vi "SimpleOscillograph.vi"() -> ()   [LabVIEW 2015]
uses:
  <vilib>/Analysis/4window.llb/Hanning Window (DBL).vi
  <vilib>/Analysis/4window.llb/Hamming Window (DBL).vi
  <vilib>/Analysis/4window.llb/Blackman Window (DBL).vi
  <vilib>/Analysis/4window.llb/Gaussian Window (DBL).vi
  <vilib>/Analysis/2dsp.llb/Real FFT.vi
  <vilib>/Analysis/4window.llb/AllCosWindow (DBL).vi
  <vilib>/Instr/_visa.llb/VISA Configure Serial Port (Serial Instr).vi
  <vilib>/Analysis/NI_AALPro.lvlib
panel:
  out "AD":i32
  out "VCC":dbl
  out "num_of_data":i32
  out "实际采样频率":dbl
  in  "采样模式":u16(ring) items=["触发", "实时"]
  in  "ABORT":bool
  in  "触发模式":u16(ring) items=["自动", "上升沿", "下降沿", "边沿"]
  in  "采 样 率":u16(ring)=3 caption="端口号" items=["100Hz", "1KHz", "10KHz", "100KHz", "250KHz", "500KHz", "1MHz"]
  in  "清空缓冲区":bool
  in  "清空波形":bool
  out "C1":dbl
  out "C2":dbl
  out "C3":dbl
  out "缓冲区字节":u32
  in  "波特率":u16(ring)=4 items=["4800", "9600", "115200", "230400", "460800"]
  out "串口状态":bool
  in  "打开串口":bool
  in  "端口号":u16(ring) items=["COM1", "COM2", "COM3", "COM4", "COM5", "COM6"]
  in  "?":enum32{"独立波形图", "混合波形图", "FFT频域图"}(tab)
  out "幅值 C3":dbl(graph)
  out "幅值 C2":dbl(graph)
  out "幅值 C1":dbl(graph)
  out "幅值":dynamicdata(graph)
  in  "FIR滤波":u16(ring) caption="端口号" items=["禁用"]
  in  "信号加窗":u16(ring) caption="端口号" items=["不加窗", "Hanning", "Hamming", "Blackman", "高斯窗"]
  in  "FFT通道":u16(ring) caption="端口号" items=["C1", "C2", "C3"]
  out "频谱图":dbl[](graph)
  out "关串口等待":u32=500
  in  "延时":u32
  out "VISA resource name":refnum<visa-resource-name> caption="VISA资源名称"
  # "SimpleOscillograph"
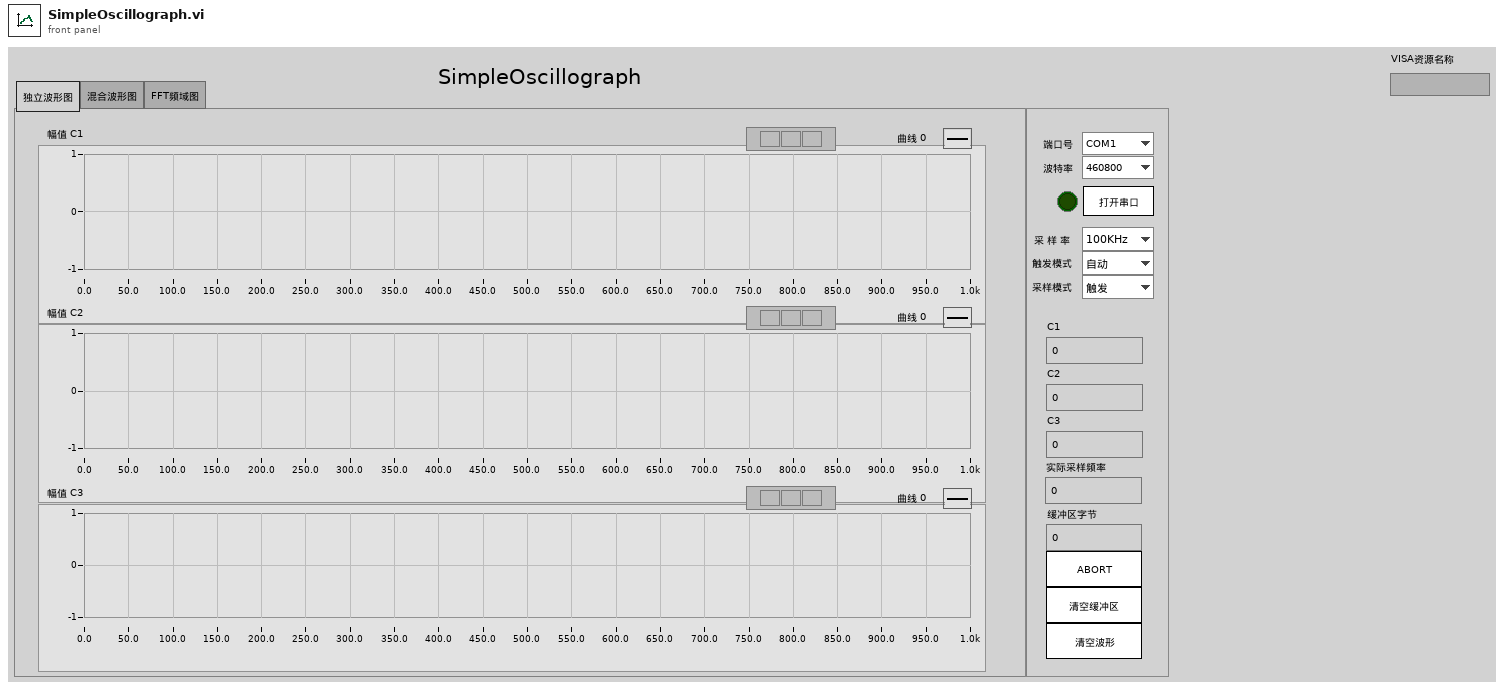
[diagram p1: front panel]
types:
  T1 = enum8{"Enabled", "Disabled", "Disabled and Grayed Out"}
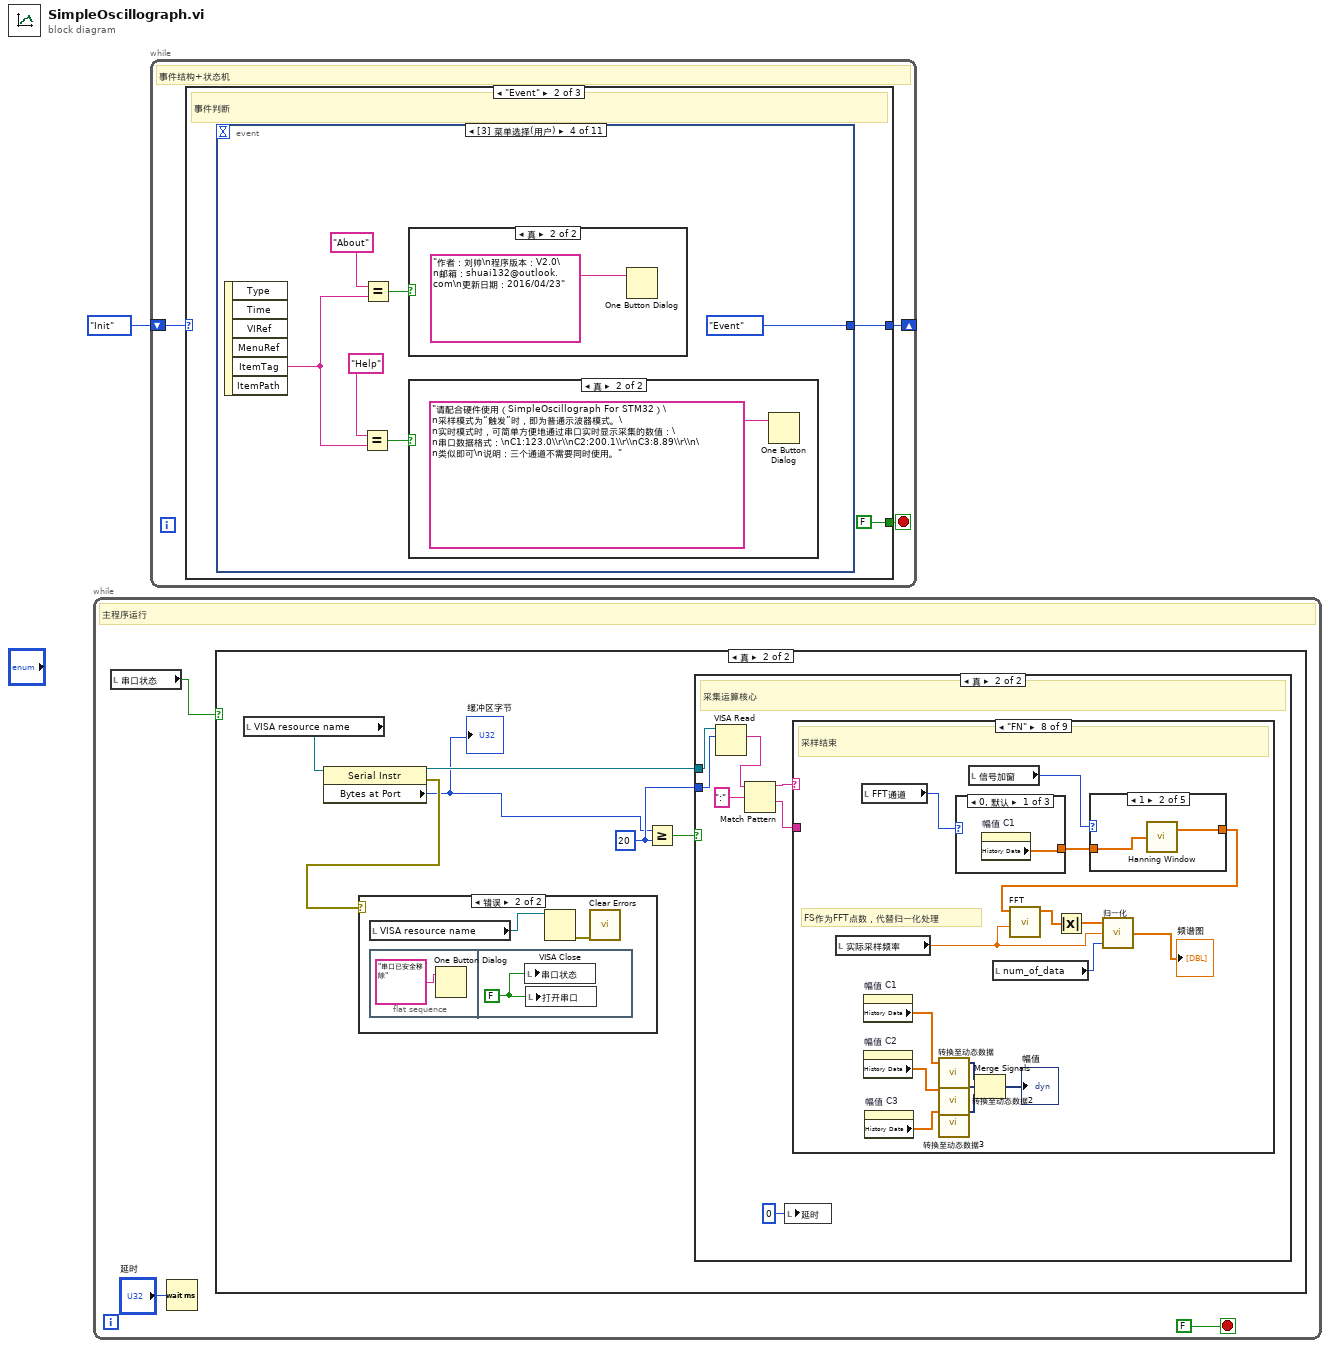
[diagram p0: block diagram]
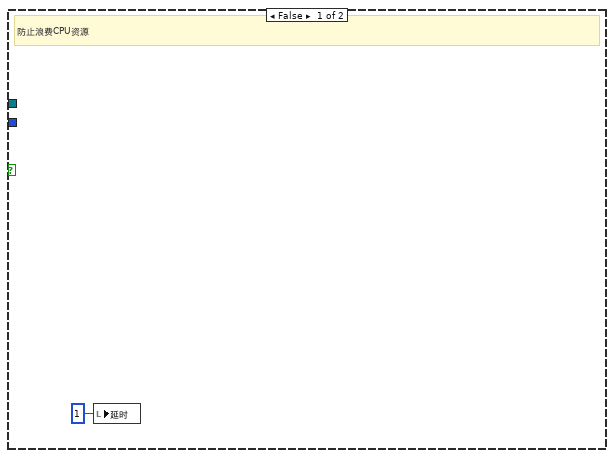
[diagram p4: hidden frame]
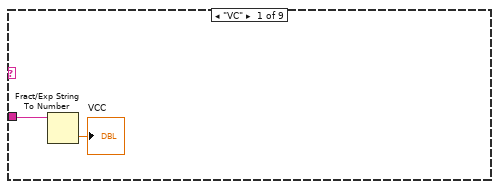
[diagram p5: hidden frame]
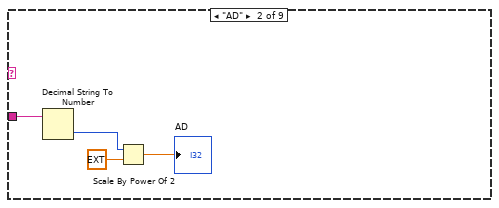
[diagram p6: hidden frame]
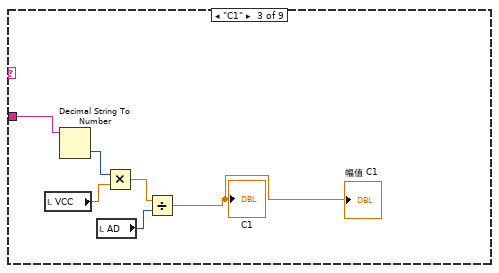
[diagram p7: hidden frame]
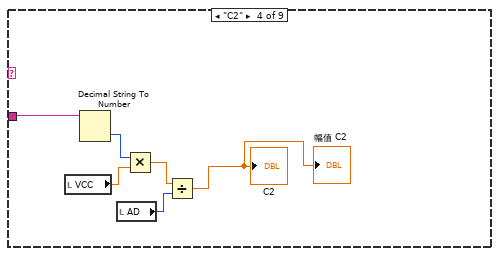
[diagram p8: hidden frame]
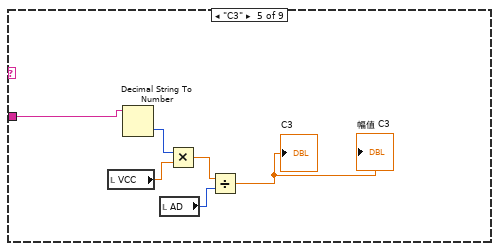
[diagram p9: hidden frame]
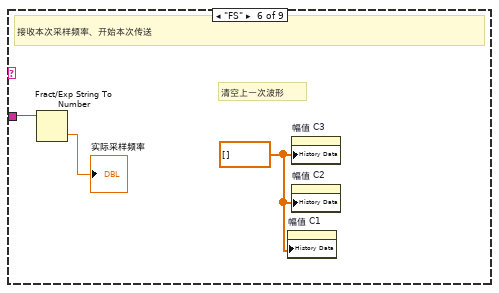
[diagram p10: hidden frame]
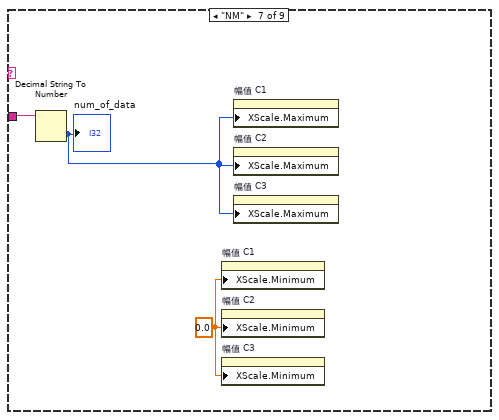
[diagram p11: hidden frame]
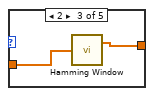
[diagram p13: hidden frame]
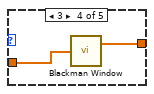
[diagram p14: hidden frame]
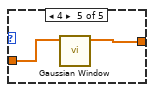
[diagram p15: hidden frame]
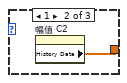
[diagram p16: hidden frame]
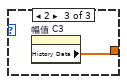
[diagram p17: hidden frame]
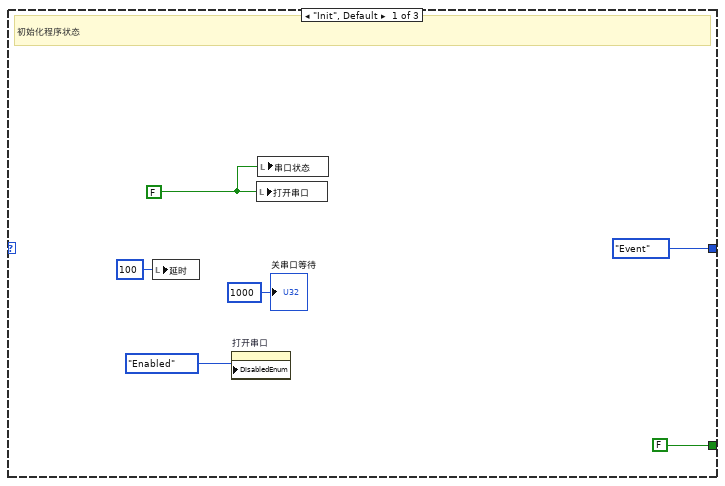
[diagram p19: hidden frame]
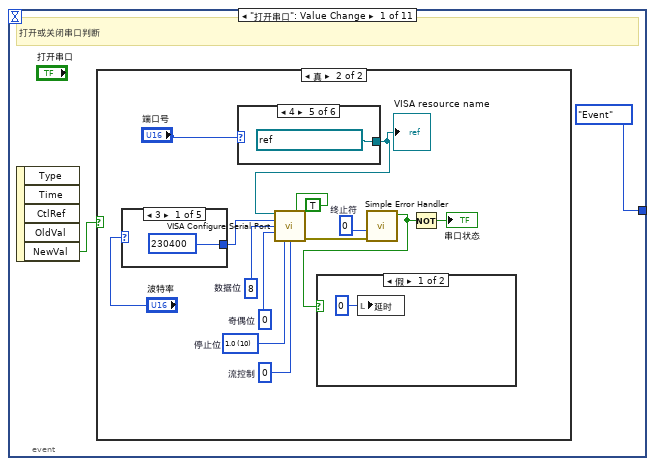
[diagram p20: hidden frame]
diagram:
  n1 = while {
    stop <- FALSE stop-if-true
    # "主程序运行"
    n2 = local read "串口状态"() -> (w4:bool)
    n3 = Wait (ms)(milliseconds to wait="延时") -> ()  [unwired: 1 out]
    n4 = case shown="真" w4 {
      frame False {
      }
      frame True {
        w6 = u32 20 ("y")
        n5 = local read "VISA resource name"() -> (w10:refnum<visa-resource-name>)
        n6 = property class="Serial Instr"(reference=w10) -> (reference out=w9:refnum<visa-resource-name>, error out=w8:errorcluster, "Bytes at Port"=w5:u32)  [unwired: 1 in]
        "缓冲区字节" <- w5
        n7 = case shown="错误" w8 {
          frame No Error {
          }
          frame Error {
            n8 = local read "VISA resource name"() -> (w11:refnum<visa-resource-name>)
            n9 = flat-sequence {
              frame #0 {
                n10 = One Button Dialog(message="串口已安全移除") -> ()  [unwired: 1 in, 1 out]
              }
              frame #1 {
                w14 = FALSE ("exit")
                n11 = local write "串口状态"(w14) -> ()
                n12 = local write "打开串口"(w14) -> ()
              }
            }
            n13 = VISA Close(VISA resource name=w11) -> (error out=w12:errorcluster)  [unwired: 1 in]
            n14 = call <vilib>:"Clear Errors.vi"("error in (no error)"=w12) -> ()  [unwired: 5 in, 2 out]
          }
        }
        n15 = Greater Or Equal?(x=w5, y=w6) -> (x >= y?=w7:bool)
        n16 = case shown="真" w7 {
          tunnel: w9 -> [_ w22]
          tunnel: w6 -> [_ w21]
          frame False {
            # "防止浪费CPU资源"
            n17 = local write "延时"(u32 1 ("延时")) -> ()
          }
          frame True {
            # "采集运算核心"
            n18 = VISA Read(VISA resource name=w22, byte count=w21) -> (read buffer=w16:string)  [unwired: 1 in, 3 out]
            n19 = Match Pattern(string=w16, regular expression=":" ("正则表达式")) -> (before substring=w18:string, after substring=w19:string)  [unwired: 1 in, 2 out]
            n20 = local write "延时"(u32 0 ("延时")) -> ()
            n21 = case shown="\"FN\"" w18 {
              tunnel: w19 -> [w24 w28 w34 w36 w42 w49 w52 _ _]
              frame "VC" {
                n22 = Fract/Exp String To Number(string=w24) -> (number=→"VCC":dbl)  [unwired: 3 in, 1 out]
              }
              frame "AD" {
                n23 = Decimal String To Number(string=w28) -> (number=w27:i32)  [unwired: 2 in, 1 out]
                n24 = Scale By Power Of 2(n=w27, x=ext 1.0) -> (x*2^n=→"AD":ext)
              }
              frame "C1" {
                n25 = local read "VCC"() -> (w32:dbl)
                n26 = Decimal String To Number(string=w34) -> (number=w33:i32)  [unwired: 2 in, 1 out]
                n27 = local read "AD"() -> (w30:i32)
                n28 = Multiply(x=w33, y=w32) -> (x*y=w31:dbl)
                n29 = Divide(x=w31, y=w30) -> (x/y=→"C1" →"幅值 C1":dbl)
              }
              frame "C2" {
                n30 = local read "VCC"() -> (w39:dbl)
                n31 = Decimal String To Number(string=w36) -> (number=w40:i32)  [unwired: 2 in, 1 out]
                n32 = local read "AD"() -> (w37:i32)
                n33 = Multiply(x=w40, y=w39) -> (x*y=w38:dbl)
                n34 = Divide(x=w38, y=w37) -> (x/y=→"C2" →"幅值 C2":dbl)
              }
              frame "C3" {
                n35 = local read "VCC"() -> (w45:dbl)
                n36 = Decimal String To Number(string=w42) -> (number=w46:i32)  [unwired: 2 in, 1 out]
                n37 = local read "AD"() -> (w43:i32)
                n38 = Multiply(x=w46, y=w45) -> (x*y=w44:dbl)
                n39 = Divide(x=w44, y=w43) -> (x/y=→"C3" →"幅值 C3":dbl)
              }
              frame "FS" {
                w47 = dbl[] [] ("历史数据")
                # "清空上一次波形"
                # "接收本次采样频率、开始本次传送"
                n40 = Fract/Exp String To Number(string=w49) -> (number=→"实际采样频率":dbl)  [unwired: 3 in, 1 out]
                n41 = property on="幅值 C1" class="WFChart (严格)"("History Data"=w47) -> ()  [unwired: 2 in, 2 out]
                n42 = property on="幅值 C3" class="WFChart (严格)"("History Data"=w47) -> ()  [unwired: 2 in, 2 out]
                n43 = property on="幅值 C2" class="WFChart (严格)"("History Data"=w47) -> ()  [unwired: 2 in, 2 out]
              }
              frame "NM" {
                w50 = 0.0 ("X标尺.范围:最小值")
                n44 = Decimal String To Number(string=w52) -> (number=w51:i32)  [unwired: 2 in, 1 out]
                "num_of_data" <- w51
                n45 = property on="幅值 C1" class="WFChart (严格)"("XScale.Minimum"=w50) -> ()  [unwired: 2 in, 2 out]
                n46 = property on="幅值 C2" class="WFChart (严格)"("XScale.Minimum"=w50) -> ()  [unwired: 2 in, 2 out]
                n47 = property on="幅值 C3" class="WFChart (严格)"("XScale.Minimum"=w50) -> ()  [unwired: 2 in, 2 out]
                n48 = property on="幅值 C1" class="WFChart (严格)"("XScale.Maximum"=w51) -> ()  [unwired: 2 in, 2 out]
                n49 = property on="幅值 C2" class="WFChart (严格)"("XScale.Maximum"=w51) -> ()  [unwired: 2 in, 2 out]
                n50 = property on="幅值 C3" class="WFChart (严格)"("XScale.Maximum"=w51) -> ()  [unwired: 2 in, 2 out]
              }
              frame "FN" {
                # "FS作为FFT点数，代替归一化处理"
                # "采样结束"
                n51 = local read "实际采样频率"() -> (w62:dbl)
                n52 = local read "FFT通道"() -> (w68:u16)
                n53 = property on="幅值 C1" class="WFChart (严格)"() -> ("History Data"=w59:dbl[])  [unwired: 2 in, 2 out]
                n54 = property on="幅值 C2" class="WFChart (严格)"() -> ("History Data"=w57:dbl[])  [unwired: 2 in, 2 out]
                n55 = property on="幅值 C3" class="WFChart (严格)"() -> ("History Data"=w55:dbl[])  [unwired: 2 in, 2 out]
                n56 = call "转换至动态数据"("Array"=w59) -> ("Dynamic Data Type"=w58:dynamicdata)  [unwired: 3 in]
                n57 = call "转换至动态数据2"("Array"=w57) -> ("Dynamic Data Type"=w56:dynamicdata)  [unwired: 3 in]
                n58 = call "转换至动态数据3"("Array"=w55) -> ("Dynamic Data Type"=w54:dynamicdata)  [unwired: 3 in]
                n59 = case shown="0, 默认" w68 {
                  tunnel: [w78 w79 w80] -> w67
                  frame 0, Default {
                    n60 = property on="幅值 C1" class="WFChart (严格)"() -> ("History Data"=w78:dbl[])  [unwired: 2 in, 2 out]
                  }
                  frame 1 {
                    n61 = property on="幅值 C2" class="WFChart (严格)"() -> ("History Data"=w79:dbl[])  [unwired: 2 in, 2 out]
                  }
                  frame 2 {
                    n62 = property on="幅值 C3" class="WFChart (严格)"() -> ("History Data"=w80:dbl[])  [unwired: 2 in, 2 out]
                  }
                }
                n63 = local read "信号加窗"() -> (w66:u16)
                n64 = Merge Signals(w58, w56, w54) -> (→"幅值":dynamicdata)
                n65 = local read "num_of_data"() -> (w60:i32)
                n66 = case shown="1" w66 {
                  tunnel: w67 -> [w69 w71 w73 w75 w77]
                  tunnel: [w69 w70 w72 w74 w76] -> w64
                  frame 0, Default {
                  }
                  frame 1 {
                    n67 = call-poly <vilib>:"Hanning Window.vi"("X"=w71) -> ("Windowed X"=w70:dbl[])  [unwired: 1 out]
                  }
                  frame 2 {
                    n68 = call-poly <vilib>:"Hamming Window.vi"("X"=w73) -> ("Windowed X"=w72:dbl[])  [unwired: 1 out]
                  }
                  frame 3 {
                    n69 = call-poly <vilib>:"Blackman Window.vi"("X"=w75) -> ("Windowed X"=w74:dbl[])  [unwired: 1 out]
                  }
                  frame 4 {
                    n70 = call-poly <vilib>:"Gaussian Window.vi"("X"=w77) -> ("Windowed X"=w76:dbl[])  [unwired: 9 in, 1 out]
                  }
                }
                n71 = call-poly <vilib>:"FFT.vi"("FFT size"=w62, "X"=w64) -> ("FFT {X}"=w65:cdb[])  [unwired: 8 in, 1 out]
                n72 = Absolute Value(x=w65) -> (abs(x)=w63:dbl[])
                n73 = call "归一化.vi"("实际参采样点数"=w60, "FFT点数"=w62, "数组输入"=w63) -> ("数组输出"=→"频谱图":dbl[])
              }
              frame Default {
              }
            }
          }
        }
      }
    }
  }
  n74 = while {
    shift-right: [w81] -> _
    shift-left: enum16{"Init", "Event", "Exit"}."Init" -> [w82]
    stop <- w83 stop-if-true
    # "事件结构+状态机"
    n75 = case shown="\"Event\"" w82 {
      tunnel: [FALSE FALSE TRUE] -> w83
      tunnel: [enum16{"Init", "Event", "Exit"}."Event" w90 enum16{"Init", "Event", "Exit"}."Exit"] -> w81
      frame "Init", Default {
        w87 = FALSE ("exit")
        # "初始化程序状态"
        n76 = local write "延时"(u32 100 ("延时")) -> ()
        n77 = property on="打开串口" class="Bool (严格)"("DisabledEnum"=T1."Enabled" ("禁用")) -> ()  [unwired: 2 in, 2 out]
        n78 = local write "打开串口"(w87) -> ()
        n79 = local write "串口状态"(w87) -> ()
        "关串口等待" <- u32 1000 ("关串口等待")
      }
      frame "Event" {
        # "事件判断"
        n80 = event shown="[3] 菜单选择(用户)" {
          selector: _ -> [_ _ _ _ _ _ _ _ _ _ _]
          dyn-events: _ -> [_ _ _ _ _ _ _ _ _ _ _]
          timeout: _ -> [_ _ _ _ _ _ _ _ _ _ _]
          tunnel: [enum16{"Init", "Event", "Exit"}."Event" enum16{"Init", "Event", "Exit"}."Event" enum16{"Init", "Event", "Exit"}."Event" enum16{"Init", "Event", "Exit"}."Event" enum16{"Init", "Event", "Exit"}."Event" enum16{"Init", "Event", "Exit"}."Event" enum16{"Init", "Event", "Exit"}."Event" enum16{"Init", "Event", "Exit"}."Event" enum16{"Init", "Event", "Exit"}."Event" enum16{"Init", "Event", "Exit"}."Event" enum16{"Init", "Event", "Exit"}."Exit"] -> w90
          event "打开串口": Value Change {
            # "打开或关闭串口判断"
            n81 = event-data() -> ("NewVal"=w92:bool)  [unwired: 1 in, 4 out]
            n82 = case shown="真" w92 {
              frame False {
                n83 = local read "串口状态"() -> (w94:bool)
                n84 = case shown="真" w94 {
                  frame False {
                  }
                  frame True {
                    # "故意先关串口状态\n这样主程序就不会占用串口了\n降低出错的可能"
                    n85 = flat-sequence {
                      frame #0 {
                        n86 = local write "串口状态"(FALSE) -> ()
                        n87 = local write "延时"(u32 100 ("延时")) -> ()
                      }
                      frame #1 {
                        n88 = local read "VISA resource name"() -> (w97:refnum<visa-resource-name>)
                        n89 = VISA Close(VISA resource name=w97) -> (error out=w98:errorcluster)  [unwired: 1 in]
                        n90 = call <vilib>:"Simple Error Handler.vi"("error in (no error)"=w98) -> ()  [unwired: 4 in, 5 out]
                      }
                      frame #2 {
                        n91 = local read "关串口等待"() -> (w99:u32)
                        n92 = Wait (ms)(milliseconds to wait=w99) -> ()  [unwired: 1 out]
                      }
                    }
                  }
                }
              }
              frame True {
                w100 = u16 10 items=["1.0"=10, "1.5"=15, "2.0"=20]  # 停止位
                w104 = TRUE  # 终止符
                w110 = u16 0  # 流控制
                w109 = u8 0  # 奇偶位
                w108 = u16 8  # 数据位
                n93 = case shown="3" "波特率" {
                  tunnel: [230400 460800 4800 9600 115200] -> w107
                  frame 3 {
                  }
                  frame 4 {
                  }
                  frame 0, Default {
                  }
                  frame 1 {
                  }
                  frame 2 {
                  }
                }
                n94 = case shown="4" "端口号" {
                  tunnel: [refnum<visa-resource-name> "ASRL1::INSTR" ("VISA resource name") refnum<visa-resource-name> "ASRL2::INSTR" ("VISA resource name") refnum<visa-resource-name> "ASRL3::INSTR" ("VISA resource name") refnum<visa-resource-name> "ASRL4::INSTR" ("VISA resource name") refnum<visa-resource-name> "ASRL5::INSTR" ("VISA resource name") refnum<visa-resource-name> "ASRL6::INSTR" ("VISA resource name")] -> w101
                  frame 0, Default {
                  }
                  frame 1 {
                  }
                  frame 2 {
                  }
                  frame 3 {
                  }
                  frame 4 {
                  }
                  frame 5 {
                  }
                }
                "VISA resource name" <- w101
                n95 = call-poly "VISA Configure Serial Port"("VISA resource name"=w101, "Enable Termination\nChar (T)"=w104, "baud rate (9600)"=w107, "data bits (8)"=w108, "parity (0:none)"=w109, "stop bits (10: 1 bit)"=w100, "flow control (0:none)"=w110) -> ("error out"=w111:errorcluster)  [unwired: 7 in, 1 out]
                n96 = call <vilib>:"Simple Error Handler.vi"("type of dialog (OK msg:1)"=0, "error in (no error)"=w111) -> ("error?"=w105:bool)  [unwired: 3 in, 4 out]
                n97 = case shown="假" w105 {
                  frame False {
                    n98 = local write "延时"(u32 0 ("延时")) -> ()
                  }
                  frame True {
                    n99 = One Button Dialog(message="串口不存在或已打开！") -> ()  [unwired: 1 in, 1 out]
                    n100 = local write "打开串口"(FALSE) -> ()
                  }
                }
                n101 = Not(x=w105) -> (.not. x?=→"串口状态":bool)
              }
            }
          }
          event "端口号", "波特率": Value Change {
            n102 = event-data() -> ("OldVal"=w128:u16)  [unwired: 1 in, 4 out]
            n103 = local read "串口状态"() -> (w129:bool)
            n104 = case shown="真" w129 {
              tunnel: w128 -> [_ w130]
              frame False {
              }
              frame True {
                n105 = flat-sequence {
                  tunnel: w130 -> [w135]
                  frame #0 {
                    n106 = case shown="0, 默认" w135 {
                      tunnel: [refnum<visa-resource-name> "ASRL1::INSTR" ("VISA resource name") refnum<visa-resource-name> "ASRL2::INSTR" ("VISA resource name") refnum<visa-resource-name> "ASRL3::INSTR" ("VISA resource name") refnum<visa-resource-name> "ASRL4::INSTR" ("VISA resource name") refnum<visa-resource-name> "ASRL5::INSTR" ("VISA resource name")] -> w132
                      frame 0, Default {
                      }
                      frame 1 {
                      }
                      frame 2 {
                      }
                      frame 3 {
                      }
                      frame 4 {
                      }
                    }
                    n107 = VISA Close(VISA resource name=w132) -> (error out=w134:errorcluster)  [unwired: 1 in]
                    n108 = call <vilib>:"Simple Error Handler.vi"("error in (no error)"=w134) -> ()  [unwired: 4 in, 5 out]
                    n109 = local write "串口状态"(FALSE) -> ()
                    n110 = local write "打开串口"(FALSE ("open")) -> ()
                  }
                }
              }
            }
          }
          event "清空缓冲区": Value Change {
            n111 = event-data() -> ()  [unwired: 1 in, 6 out]
            n112 = local read "串口状态"() -> (w141:bool)
            n113 = case shown="真" w141 {
              frame False {
                n114 = call "显示对话框信息"() -> ()  [unwired: 10 in, 2 out]
              }
              frame True {
                n115 = local read "VISA resource name"() -> (w143:refnum<visa-resource-name>)
                n116 = VISA Flush I/O Buffer(VISA resource name=w143) -> ()  [unwired: 2 in, 2 out]
              }
            }
          }
          event Menu Selection (User) {
            n117 = event-data() -> ("ItemTag"=w147:string)  [unwired: 1 in, 5 out]
            n118 = Equal?(x="Help", y=w147) -> (x = y?=w148:bool)
            n119 = Equal?(x="About", y=w147) -> (x = y?=w149:bool)
            n120 = case shown="真" w149 {
              frame False {
              }
              frame True {
                n121 = One Button Dialog(message="作者：刘帅\n程序版本：V2.0\n邮箱：shuai132@outlook.com\n更新日期：2016/04/23" ("Message")) -> ()  [unwired: 1 in, 1 out]
              }
            }
            n122 = case shown="真" w148 {
              frame False {
              }
              frame True {
                n123 = One Button Dialog(message="请配合硬件使用（SimpleOscillograph For STM32）\n采样模式为“触发”时，即为普通示波器模式。\n实时模式时，可简单方便地通过串口实时显示采集的数值：\n串口数据格式：\nC1:123.0\\r\\nC2:200.1\\r\\nC3:8.89\\r\\n\n类似即可\n说明：三个通道不需要同时使用。" ("Message")) -> ()  [unwired: 1 in, 1 out]
              }
            }
          }
          event "清空波形": Value Change {
            w152 = dbl[] [] ("历史数据")
            n124 = event-data() -> ()  [unwired: 1 in, 6 out]
            n125 = property on="幅值 C3" class="WFChart (严格)"("History Data"=w152) -> ()  [unwired: 2 in, 2 out]
            n126 = property on="幅值 C2" class="WFChart (严格)"("History Data"=w152) -> ()  [unwired: 2 in, 2 out]
            n127 = property on="幅值 C1" class="WFChart (严格)"("History Data"=w152) -> ()  [unwired: 2 in, 2 out]
            n128 = property on="幅值" class="WFChart (严格)"("History Data"=dynamicdata[] [] ("历史数据")) -> ()  [unwired: 2 in, 2 out]
          }
          event "采 样 率": Value Change; "采 样 率": Mouse Down {
            n129 = event-data() -> ()  [unwired: 1 in, 4 out]
            n130 = local read "串口状态"() -> (w156:bool)
            n131 = case shown="真" w156 {
              frame False {
                n132 = call "显示对话框信息2"() -> ()  [unwired: 10 in, 2 out]
              }
              frame True {
                n133 = Number To Decimal String(number="采 样 率") -> (decimal integer string=w158:string)  [unwired: 1 in]
                n134 = local read "VISA resource name"() -> (w160:refnum<visa-resource-name>)
                n135 = Concatenate Strings("FS:" ("字符串"), w158, " " ("字符串")) -> (w162:string)
                n136 = VISA Write(VISA resource name=w160, write buffer=w162) -> ()  [unwired: 1 in, 3 out]
              }
            }
          }
          event "触发模式": Value Change; "触发模式": Mouse Down {
            n137 = event-data() -> ()  [unwired: 1 in, 4 out]
            n138 = local read "串口状态"() -> (w164:bool)
            n139 = case shown="真" w164 {
              frame False {
                n140 = call "显示对话框信息3"() -> ()  [unwired: 10 in, 2 out]
              }
              frame True {
                # "Trigger mode"
                n141 = Number To Decimal String(number="触发模式") -> (decimal integer string=w166:string)  [unwired: 1 in]
                n142 = local read "VISA resource name"() -> (w168:refnum<visa-resource-name>)
                n143 = Concatenate Strings("TM:" ("字符串"), w166, " " ("字符串")) -> (w170:string)
                n144 = VISA Write(VISA resource name=w168, write buffer=w170) -> ()  [unwired: 1 in, 3 out]
              }
            }
          }
          event "ABORT": Value Change {
            w171 = dbl[] [] ("历史数据")
            n145 = event-data() -> ()  [unwired: 1 in, 6 out]
            n146 = property on="幅值 C3" class="WFChart (严格)"("History Data"=w171) -> ()  [unwired: 2 in, 2 out]
            n147 = property on="幅值 C2" class="WFChart (严格)"("History Data"=w171) -> ()  [unwired: 2 in, 2 out]
            n148 = property on="幅值 C1" class="WFChart (严格)"("History Data"=w171) -> ()  [unwired: 2 in, 2 out]
            n149 = local read "串口状态"() -> (w173:bool)
            n150 = property on="幅值" class="WFChart (严格)"("History Data"=dynamicdata[] [] ("历史数据")) -> ()  [unwired: 2 in, 2 out]
            n151 = case shown="真" w173 {
              frame False {
                n152 = call "显示对话框信息4"() -> ()  [unwired: 10 in, 2 out]
              }
              frame True {
                # "ABORT"
                n153 = local read "VISA resource name"() -> (w176:refnum<visa-resource-name>)
                n154 = VISA Write(VISA resource name=w176, write buffer="AB:1 " ("字符串")) -> ()  [unwired: 1 in, 3 out]
              }
            }
          }
          event "采样模式": Value Change; "采样模式": Mouse Down {
            n155 = event-data() -> ()  [unwired: 1 in, 4 out]
            n156 = local read "串口状态"() -> (w178:bool)
            n157 = case shown="真" w178 {
              frame False {
                n158 = call "显示对话框信息5"() -> ()  [unwired: 10 in, 2 out]
              }
              frame True {
                n159 = property on="幅值 C1" class="WFChart (严格)"("ActXScl"=0 ("活动X标尺")) -> ()  [unwired: 2 in, 2 out]
                n160 = Number To Decimal String(number="采样模式") -> (decimal integer string=w183:string)  [unwired: 1 in]
                n161 = local read "VISA resource name"() -> (w185:refnum<visa-resource-name>)
                n162 = Concatenate Strings("SM:" ("字符串"), w183, " " ("字符串")) -> (w182:string)
                n163 = VISA Write(VISA resource name=w185, write buffer=w182) -> ()  [unwired: 1 in, 3 out]
              }
            }
          }
          event "FFT通道", "信号加窗", "FIR滤波": Value Change; "FFT通道": Key Down; "信号加窗", "FIR滤波": Mouse Down {
            # "FS作为FFT点数，归一化处理"
            n164 = event-data() -> ()  [unwired: 1 in, 4 out]
            n165 = case shown="0, 默认" "FFT通道" {
              tunnel: [w205 w206 w207] -> w191
              frame 0, Default {
                n166 = property on="幅值 C1" class="WFChart (严格)"() -> ("History Data"=w205:dbl[])  [unwired: 2 in, 2 out]
              }
              frame 1 {
                n167 = property on="幅值 C2" class="WFChart (严格)"() -> ("History Data"=w206:dbl[])  [unwired: 2 in, 2 out]
              }
              frame 2 {
                n168 = property on="幅值 C3" class="WFChart (严格)"() -> ("History Data"=w207:dbl[])  [unwired: 2 in, 2 out]
              }
            }
            n169 = local read "实际采样频率"() -> (w186:dbl)
            n170 = case shown="1" "信号加窗" {
              tunnel: w191 -> [w196 w198 w200 w202 w204]
              tunnel: [w196 w197 w199 w201 w203] -> w193
              frame 0, Default {
              }
              frame 1 {
                n171 = call-poly <vilib>:"Hanning Window.vi"("X"=w198) -> ("Windowed X"=w197:dbl[])  [unwired: 1 out]
              }
              frame 2 {
                n172 = call-poly <vilib>:"Hamming Window.vi"("X"=w200) -> ("Windowed X"=w199:dbl[])  [unwired: 1 out]
              }
              frame 3 {
                n173 = call-poly <vilib>:"Blackman Window.vi"("X"=w202) -> ("Windowed X"=w201:dbl[])  [unwired: 1 out]
              }
              frame 4 {
                n174 = call-poly <vilib>:"Gaussian Window.vi"("X"=w204) -> ("Windowed X"=w203:dbl[])  [unwired: 9 in, 1 out]
              }
            }
            n175 = local read "num_of_data"() -> (w187:i32)
            n176 = call-poly <vilib>:"FFT.vi"("FFT size"=w186, "X"=w193) -> ("FFT {X}"=w195:cdb[])  [unwired: 8 in, 1 out]
            n177 = Absolute Value(x=w195) -> (abs(x)=w189:dbl[])
            n178 = call "归一化.vi"("实际参采样点数"=w187, "FFT点数"=w186, "数组输入"=w189) -> ("数组输出"=w188:dbl[])
            n179 = local write "频谱图"(w188) -> ()
          }
          event Application Instance Close {
            # "退出程序"
            n180 = event-data() -> ()  [unwired: 1 in, 4 out]
            n181 = local read "串口状态"() -> (w209:bool)
            n182 = case shown="真" w209 {
              frame False {
              }
              frame True {
                # "故意先关串口状态\n这样主程序就不会占用串口了\n降低出错的可能"
                n183 = flat-sequence {
                  frame #0 {
                    n184 = local write "串口状态"(FALSE) -> ()
                    n185 = local write "延时"(u32 100 ("延时")) -> ()
                  }
                  frame #1 {
                    n186 = local read "VISA resource name"() -> (w212:refnum<visa-resource-name>)
                    n187 = VISA Close(VISA resource name=w212) -> (error out=w213:errorcluster)  [unwired: 1 in]
                    n188 = call <vilib>:"Simple Error Handler.vi"("error in (no error)"=w213) -> ()  [unwired: 4 in, 5 out]
                  }
                  frame #2 {
                    n189 = local read "关串口等待"() -> (w214:u32)
                    n190 = Wait (ms)(milliseconds to wait=w214) -> ()  [unwired: 1 out]
                  }
                }
              }
            }
          }
        }
      }
      frame "Exit" {
        # "退出前要处理的内容"
      }
    }
  }
